vi "GT_StartDouble.vi"(2 "mask":i16, 3 "rtn_In":cluster{"rtn":i16, "Func":string}) -> (1 "rtn_Out":cluster{"rtn":i16, "Func":string})   [LabVIEW 2014]
uses:
  VC6/gts.dll
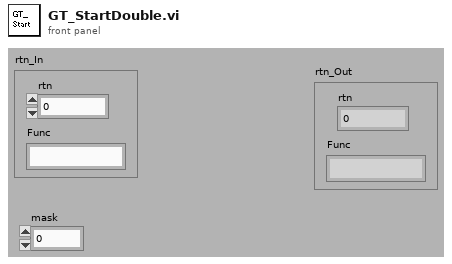
[diagram p1: front panel]
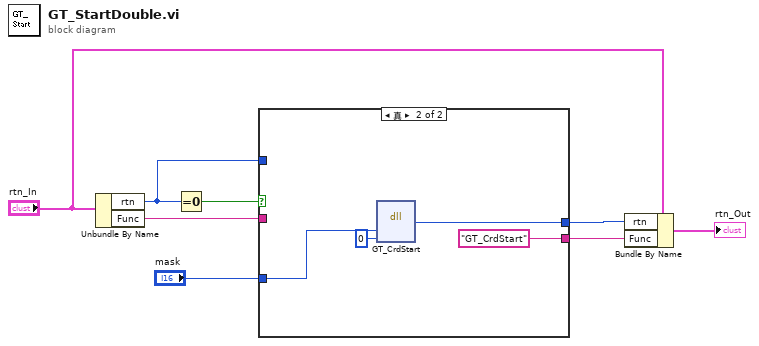
[diagram p0: block diagram]
diagram:
  n1 = Unbundle By Name("rtn_In") -> ("rtn"=w2:i16, "Func"=w1:string)
  n2 = Equal To 0?(x=w2) -> (x = 0?=w8:bool)
  n3 = case shown="真" w8 {
    tunnel: [w10 w14] -> w6
    tunnel: [w9 "GT_CrdStart" ("Func")] -> w5
    tunnel: "mask" -> [_ w12]
    tunnel: w2 -> [w10 _]
    tunnel: w1 -> [w9 _]
    frame False {
    }
    frame True {
      n4 = dll-call lib="PTH2Fabs DNewGTS AC-800LWin7版源程序-20170926gts85VC6gts.dll" fn="GT_CrdStart"("mask"=w12, "Option"=i16 0) -> ("rtn"=w14:i16)  [unwired: 5 in, 2 out]
    }
  }
  n5 = Bundle By Name(cluster="rtn_In", "rtn"=w6, "Func"=w5) -> (→"rtn_Out":cluster{"rtn":i16, "Func":string})
